vi "New Configured Task.vi"(0 "channel table":T3[](array[typedef]) {"input terminal configuration" items=["default"=-1, "RSE"=10083, "NRSE"=10078, "Differential"=10106, "Pseudodifferential"=12529]; "Channel Type" items=["Voltage (V)"=0, "Charge (C)"=9, "-"=99, "SPL (Pa)"=3, "Force (lbf)"=6, "Force (N)"=1, "Acceleration (g) - IEPE"=2, "Acceleration (g) - Charge"=12, "Acceleration (g) - 4 wire DC Voltage"=22, "Velocity (in/s)"=7, "Velocity (mm/s)"=8, "Prox Probe (mil)"=4, "Prox Probe (mm)"=5]}, 1 "sample mode":i32(ring)=10123 items=["Finite Samples"=10178, "Continuous Samples"=10123, "Hardware Timed Single Point"=12522], 2 "block size":i32, 5 "sample rate":dbl, 11 "error in":errorcluster, 12 "analog reference trigger configuration":T2 {"level trigger configuration"."hysteresis" format="%.2p"; "level trigger configuration"."slope" items=["Falling", "Rising"]; "level trigger configuration"."level" format="%.2p"}) -> (4 "DAQmx analog input task":refnum<k21>, 6 "actual sample rate":dbl, 15 "error out":errorcluster)   [LabVIEW 2024, in "Dynamic Signal Acquisition (Interactive) UI.lvlib"]
doc: "Creates a new task, adds channels, sets timing, verifies, and sets SV attributes for triggering and sensors."
uses:
  Dynamic Signal Acquisition (Interactive) UI.lvlib
  <vilib>/addons/_NISVFA/_Shared subVIs/Controls/svc_Analog Level Trigger Configuration.ctl
  SFPDAQmx Channel Info.ctl
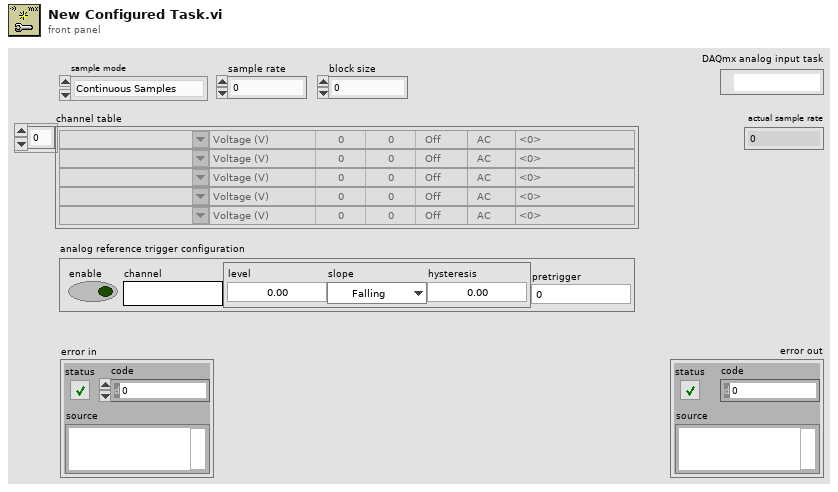
[diagram p1: front panel]
types:
  T1 = typedef "svc_Analog Level Trigger Configuration.ctl" = cluster{"level":dbl, "slope":u16, "hysteresis":dbl}
  T2 = cluster{"enable":bool, "channel":string, "level trigger configuration":T1, "pretrigger":i32}
  T3 = typedef "Dynamic Signal Acquisition (Interactive) UI.lvlib/SFPDAQmx Channel Info.ctl" = cluster{"Initialized?":bool, "DAQmx Channel":tag, "Channel Type":u16, "Max":dbl, "Sensitivity":dbl, "Excitation":bool, "Coupling":enum16{"AC", "DC"}, "input terminal configuration":i32, "excitation":enum16{"Off", "Min", "Max"}}
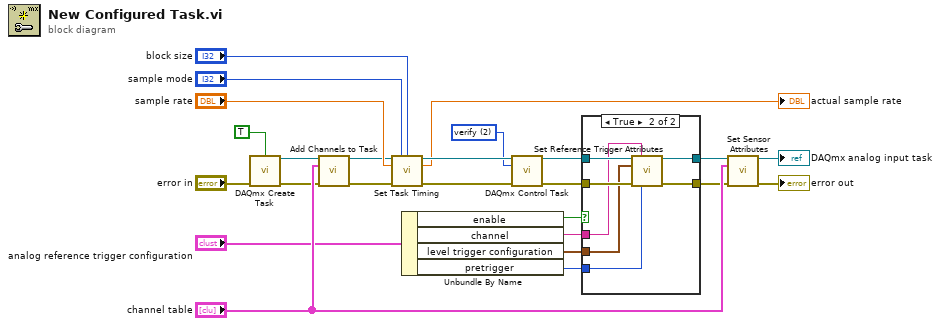
[diagram p0: block diagram]
diagram:
  w16 = 2 items=["verify"=2, "reserve"=4, "commit"=3, "unreserve"=5, "abort"=6] ("action")
  n1 = call <vilib>:"DAQmx Create Task.vi"("auto cleanup"=TRUE, "error in"="error in") -> ("task out"=w9:refnum<k21>, "error out"=w8:errorcluster)  [unwired: 12 in]
  n2 = call "Add Channels to Task.vi"("task in"=w9, "channel table"="channel table", "error in"=w8) -> ("task out"=w11:refnum<k21>, "error out"=w10:errorcluster)  [unwired: 11 in]
  n3 = call "Set Task Timing.vi"("task in"=w11, "sample mode"="sample mode", "block size"="block size", "sample rate"="sample rate", "error in"=w10) -> ("task out"=w17:refnum<k21>, "actual sample rate"=→"actual sample rate":dbl, "error out"=w18:errorcluster)  [unwired: 8 in]
  n4 = Unbundle By Name("analog reference trigger configuration") -> ("enable"=w4:bool, "channel"=w3:string, "level trigger configuration"=w2:T1, "pretrigger"=w1:i32)
  n5 = call <vilib>:"DAQmx Control Task.vi"("task/channels in"=w17, "action"=w16, "error in"=w18) -> ("task out"=w21:refnum<k21>, "error out"=w23:errorcluster)  [unwired: 11 in]
  n6 = case shown="True" w4 {
    tunnel: w21 -> [w26 w34]
    tunnel: w1 -> [_ w33]
    tunnel: w23 -> [w27 w32]
    tunnel: [w26 w31] -> w19
    tunnel: [w27 w30] -> w20
    tunnel: w3 -> [_ w29]
    tunnel: w2 -> [_ w28]
    frame False {
      # "NO Trigger"
    }
    frame True {
      n7 = call "Set Reference Trigger Attributes.vi"("task in"=w34, "trigger channel name"=w29, "level trigger configuration"=w28, "error in"=w32, "pretrigger samples"=w33) -> ("task out"=w31:refnum<k21>, "error out"=w30:errorcluster)  [unwired: 9 in]
    }
  }
  n8 = call "Set Sensor Attributes.vi"("task in"=w19, "channel table"="channel table", "error in"=w20) -> ("task out"=→"DAQmx analog input task":refnum<k21>, "error out"=→"error out":errorcluster)  [unwired: 11 in]
